vi "Write Port.vi"(8 "error in":errorcluster, 10 "port":u16, 11 "TCP master in":refnum<class "TCP Master.lvclass">) -> (0 "error out":errorcluster, 3 "TCP master out":refnum<class "TCP Master.lvclass">)   [LabVIEW 2012, in "TCP Master.lvclass"]
doc: "Property accessor for the TCP port."
uses:
  TCP Master.lvclass
  TCP Master.lvclass/TCP Master.ctl
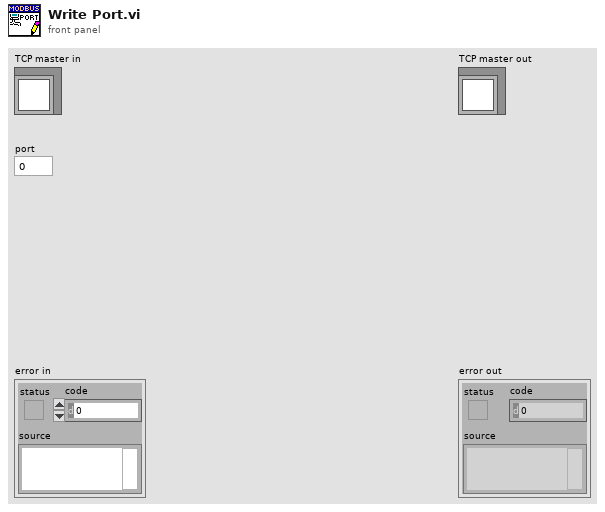
[diagram p1: front panel]
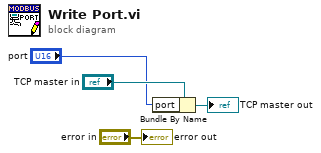
[diagram p0: block diagram]
diagram:
  n1 = Bundle By Name(cluster="TCP master in", "port"="port") -> (→"TCP master out":refnum<class "TCP Master.lvclass">)
  "error out" <- "error in"
